vi "detector choice test.vi"() -> ()   [LabVIEW 2013]
panel:
  out "String":string
  in  "number 2":i32
  in  "number":i32
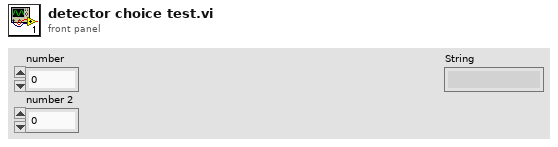
[diagram p1: front panel]
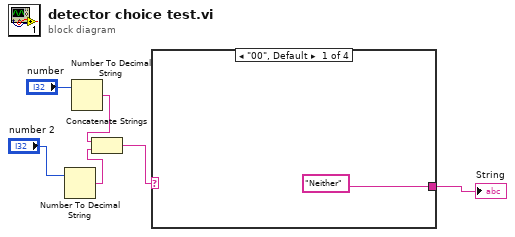
[diagram p0: block diagram]
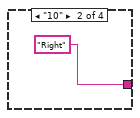
[diagram p2: hidden frame]
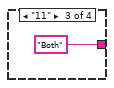
[diagram p3: hidden frame]
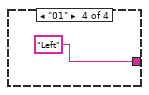
[diagram p4: hidden frame]
diagram:
  n1 = Number To Decimal String(number="number 2") -> (decimal integer string=w6:string)  [unwired: 1 in]
  n2 = Number To Decimal String(number="number") -> (decimal integer string=w5:string)  [unwired: 1 in]
  n3 = Concatenate Strings(w5, w6) -> (w4:string)
  n4 = case shown="\"00\", Default" w4 {
    tunnel: ["Neither" "Right" "Both" "Left"] -> w1
    frame "00", Default {
    }
    frame "10" {
    }
    frame "11" {
    }
    frame "01" {
    }
  }
  "String" <- w1
